vi "Decode PNG Header Chunk.vi"(10 "error in (no error)":errorcluster, 11 "data":u8[](array[numeric])) -> (2 "error out":errorcluster, 3 "Header":T1)   [LabVIEW 2021, in "Files.lvlib"]
uses:
  Files.lvlib
  PNG Header.ctl
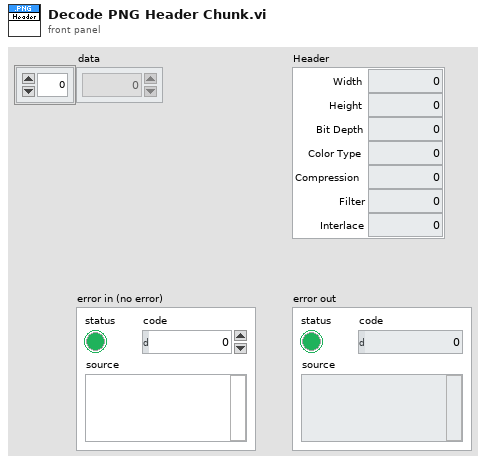
[diagram p1: front panel]
types:
  T1 = typedef "Files.lvlib/PNG Header.ctl" = cluster{"Width":u32, "Height":u32, "Bit Depth":u8, "Color Type":u8, "Compression":u8, "Filter":u8, "Interlace":u8}
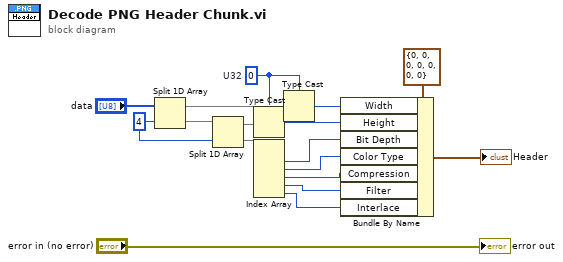
[diagram p0: block diagram]
diagram:
  w8 = u32 0  # U32
  w12 = 4 ("index")
  n1 = Split 1D Array(array="data", index=w12) -> (first subarray=w11:u8[], second subarray=w13:u8[])
  n2 = Split 1D Array(array=w13, index=w12) -> (first subarray=w9:u8[], second subarray=w6:u8[])
  n3 = Type Cast(type=w8, x=w9) -> (*(type *) &x=w7:u32)
  n4 = Index Array(array=w6) -> (element #1=w5:u8, element #2=w4:u8, element #3=w3:u8, element #4=w2:u8, element #5=w1:u8)  [unwired: 5 in]
  n5 = Type Cast(type=w8, x=w11) -> (*(type *) &x=w10:u32)
  n6 = Bundle By Name(cluster=T1 {"Width"=0, "Height"=0, "Bit Depth"=0, "Color Type"=0, "Compression"=0, "Filter"=0, "Interlace"=0} ("Header"), "Width"=w10, "Height"=w7, "Bit Depth"=w5, "Color Type"=w4, "Compression"=w3, "Filter"=w2, "Interlace"=w1) -> (→"Header":T1)
  "error out" <- "error in (no error)"
